vi "setCurrentTrack.vi"(8 "error in (no error)":errorcluster, 10 "currentTrack":u32, 11 "Player in":refnum<class "Player.lvclass">) -> (0 "error out":errorcluster, 3 "Player out":refnum<class "Player.lvclass">)   [LabVIEW 2018, in "Player.lvclass"]
uses:
  Player.lvclass
  Player.lvclass/Player.ctl
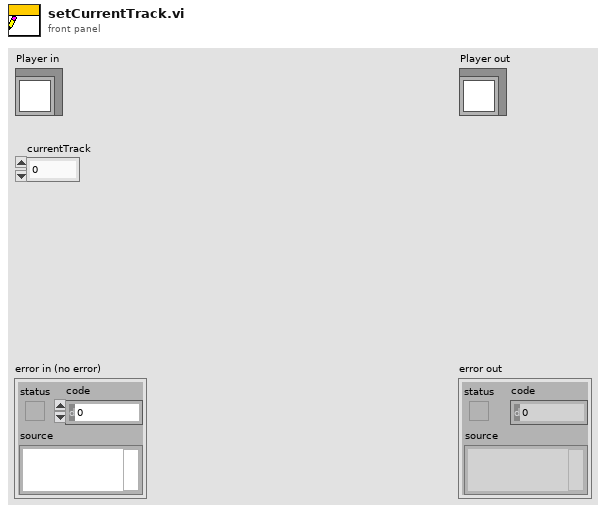
[diagram p1: front panel]
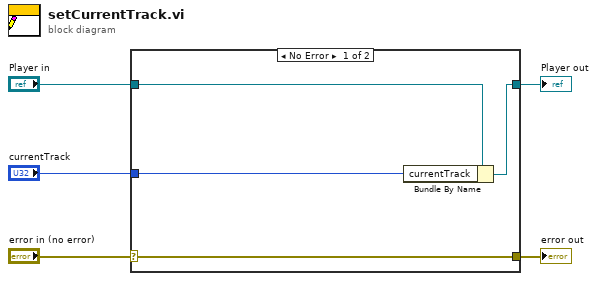
[diagram p0: block diagram]
diagram:
  n1 = case shown="No Error" "error in (no error)" {
    selector: "error in (no error)" -> [w9 w10]
    tunnel: [w9 w10] -> w4
    tunnel: [w7 w11] -> w2
    tunnel: "Player in" -> [w8 w11]
    tunnel: "currentTrack" -> [w6 _]
    frame No Error {
      n2 = Bundle By Name(cluster=w8, "currentTrack"=w6) -> (w7:refnum<class "Player.lvclass">)
    }
    frame Error {
    }
  }
  "error out" <- w4
  "Player out" <- w2
